vi "Get configuration chain.vi"(8 "error in (no error)":errorcluster, 11 "Test_ExampleClassA in":refnum<class "Test_ExampleClassA.lvclass">) -> (0 "error out":errorcluster, 1 "class name":string[](array[string]), 2 "configuration chain":variant[](array[variant]), 3 "Test_ExampleClassA out":refnum<class "Test_ExampleClassA.lvclass">)   [LabVIEW 2012, in "Test_ExampleClassA.lvclass"]
doc: "Returns an array of variants containing the configuration clusters of each class in the inheritance chain (lowest child class first), together with an array of all class names in the inheritance chain.\n\nFor classes without configuration cluster, the configuration chain contains empty variants."
uses:
  Test_ExampleClassA.lvclass
  MurmexTest/MurmexTest.lvclass
  Murmex/Murmex.lvclass
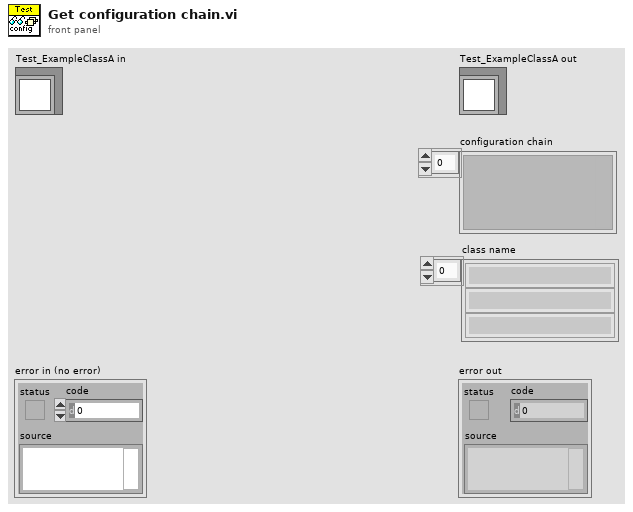
[diagram p1: front panel]
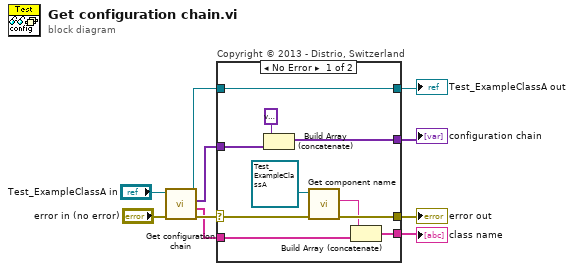
[diagram p0: block diagram]
diagram:
  n1 = call-parent "Get configuration chain.vi"("error in (no error)"="error in (no error)", "MurmexTest in"="Test_ExampleClassA in") -> ("error out"=w8:errorcluster, "class name"=w6:string[], "configuration chain"=w5:variant[], "MurmexTest out"=w7:refnum<class "Test_ExampleClassA.lvclass">)  [unwired: 6 in]
  n2 = case "Copyright © 2013 - Distrio, Switzerland" shown="No Error" w8 {
    selector: w8 -> [w19 w22]
    tunnel: [w20 w22] -> w3
    tunnel: [w17 _] -> w1
    tunnel: [w16 _] -> w2
    tunnel: [w11 w21] -> w4
    tunnel: w7 -> [w11 w21]
    tunnel: w5 -> [w14 _]
    tunnel: w6 -> [w15 _]
    frame No Error {
      n3 = Build Array (concatenate)(variant ("variant"), w14) -> (w16:variant[])
      n4 = call "Get component name.vi"("error in (no error)"=w19, "Murmex in"=refnum<class "Test_ExampleClassA.lvclass"> refnum ("Test_ExampleClassA.lvclass")) -> ("error out"=w20:errorcluster, "component name"=w18:string)  [unwired: 7 in, 1 out]
      n5 = Build Array (concatenate)(w18, w15) -> (w17:string[])
    }
    frame Error {
    }
  }
  "error out" <- w3
  "Test_ExampleClassA out" <- w4
  "configuration chain" <- w2
  "class name" <- w1
